vi "Get Result.vi"(8 "error in (no error)":errorcluster, 11 "Cryo-Con Driver in":refnum<class "Cryo-Con Driver.lvclass">) -> (0 "error out":errorcluster, 2 "Result":refnum<class "Acquired Result.lvclass">, 3 "Cryo-Con Driver out":refnum<class "Cryo-Con Driver.lvclass">)   [LabVIEW 2015, in "Cryo-Con Driver.lvclass"]
uses:
  Cryo-Con Driver.lvclass
  Measure_core/Results/Acquired Result/Acquired Result.lvclass
  VISA Instrument/VISA Instrument.lvclass/VISA Instrument.ctl
  Instrument Driver/Instrument Driver.lvclass/Instrument Driver.ctl
  <vilib>/express/express signal manip/GetorSetDDTAttributes/Shared VIs/TimeType.ctl
  Measure_core/Results/Acquired Result/Acquired Result.lvclass/Acquired Result.ctl
  VISA Instrument/Read VISA resource.vi
  Instrument Driver/Read Recorder name.vi
  VISA Instrument/Write VISA resource.vi
  Measure_core/Results/Acquired Result/Write Channels.vi
  <vilib>/express/express signal manip/GetorSetDDTAttributes/Shared VIs/TimeMode Enum to Boolean.vi
  <vilib>/express/express shared/transition.llb/Dynamic To Waveform Array.vi
  <vilib>/express/express signal manip/GetorSetDDTAttributes/Set DDT Attributes/SetT0.vi
  <vilib>/express/express shared/transition.llb/Waveform Array To Dynamic.vi
  <vilib>/express/express signal manip/GetorSetDDTAttributes/Set DDT Attributes/Set DDT Properties.xnode
  <vilib>/express/express signal manip/GetorSetDDTAttributes/Shared VIs/GetSetShared.lvlib
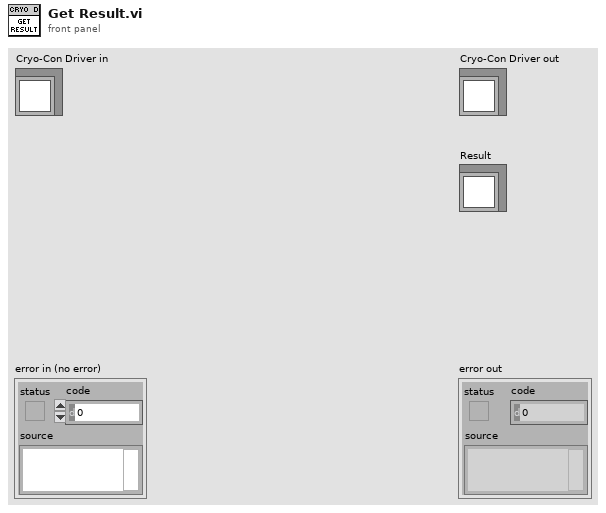
[diagram p1: front panel]
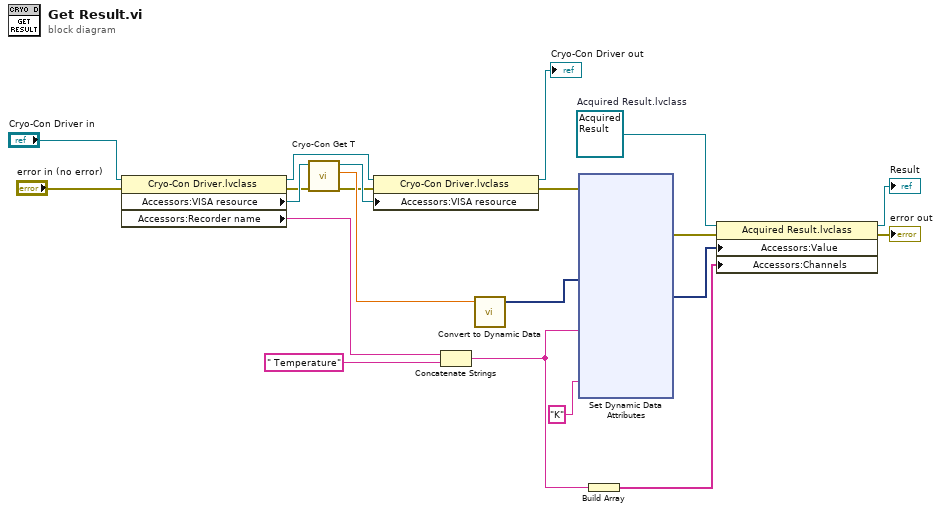
[diagram p0: block diagram]
diagram:
  w14 = refnum<class "Acquired Result.lvclass"> refnum  # Acquired Result.lvclass
  n1 = property class="Cryo-Con Driver.lvclass"(reference="Cryo-Con Driver in", error in="error in (no error)") -> (reference out=w8:refnum<class "Cryo-Con Driver.lvclass">, error out=w19:errorcluster, "Accessors:VISA resource"=w20:refnum<visa-resource-name>, "Accessors:Recorder name"=w2:string)
  n2 = call "Cryo-Con Get T.vi"("error in (no error)"=w19, "VISA Resource Name"=w20) -> ("error out"=w9:errorcluster, "Temperature"=w13:dbl, "VISA Resource Name Out"=w18:refnum<visa-resource-name>)  [unwired: 6 in, 1 out]
  n3 = property class="Cryo-Con Driver.lvclass"(reference=w8, error in=w9, "Accessors:VISA resource"=w18) -> (reference out=→"Cryo-Con Driver out":refnum<class "Cryo-Con Driver.lvclass">, error out=w6:errorcluster)
  n4 = Concatenate Strings(w2, " Temperature" ("String")) -> (w3:string)
  n5 = call "Convert to Dynamic Data"("Double"=w13) -> ("Dynamic Data Type"=w15:dynamicdata)  [unwired: 3 in]
  n6 = xnode "Set Dynamic Data Attributes"("Signals In"=w15, "Signal Name"=w3, "Unit"="K", "error in"=w6) -> ("Signals Out"=w16:dynamicdata, "error out"=w10:errorcluster)  [unwired: 3 in]
  n7 = Build Array(w3) -> (w11:string[])
  n8 = property class="Acquired Result.lvclass"(reference=w14, error in=w10, "Accessors:Value"=w16, "Accessors:Channels"=w11) -> (reference out=→"Result":refnum<class "Acquired Result.lvclass">, error out=→"error out":errorcluster)
